vi "mod.Basic1.vi"(8 "error in":errorcluster, 11 "Call Data":T1) -> (0 "error out":errorcluster, 3 "Return Data":variant)   [LabVIEW 2014]
uses:
  Private/Class/typedef.LVCallData.ctl
  Private/Class/class.GLue.lvclass
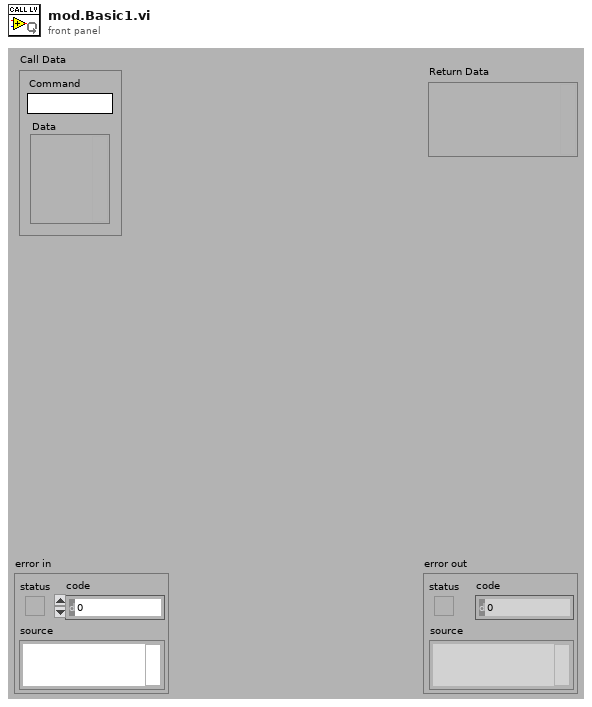
[diagram p1: front panel]
types:
  T1 = typedef "GLue.lvlib/class.GLue.lvclass/typedef.LVCallData.ctl" = cluster{"Command":string, "Data":variant}
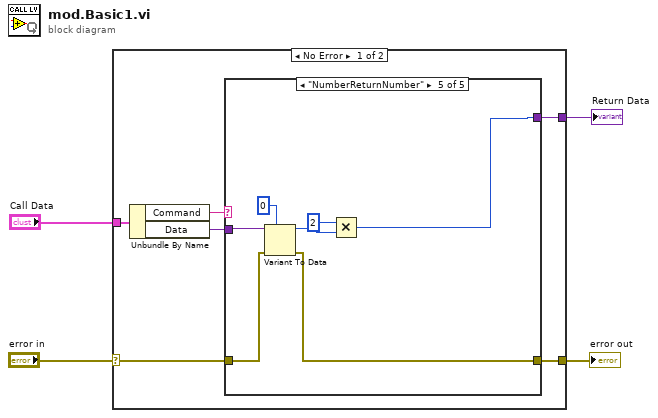
[diagram p0: block diagram]
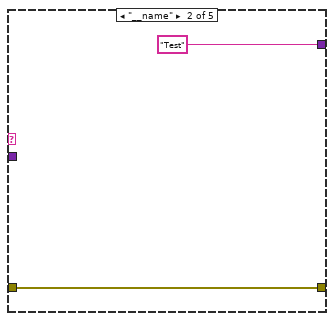
[diagram p3: hidden frame]
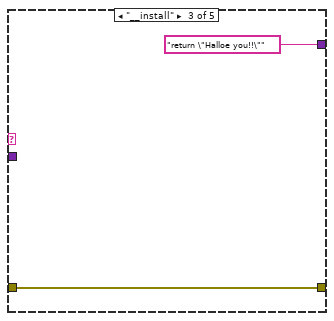
[diagram p4: hidden frame]
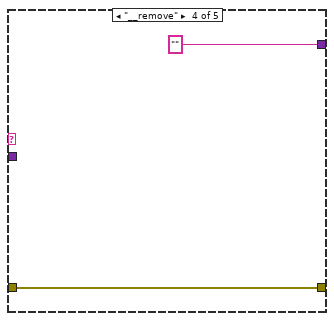
[diagram p5: hidden frame]
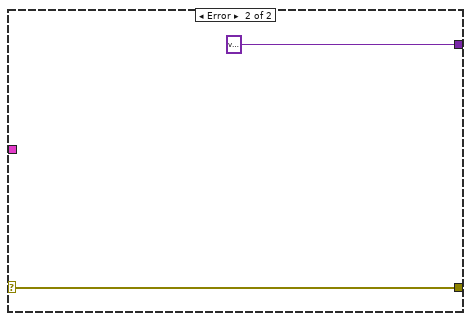
[diagram p6: hidden frame]
diagram:
  n1 = case shown="No Error" "error in" {
    selector: "error in" -> [w9 w27]
    tunnel: [w5 w27] -> w3
    tunnel: "Call Data" -> [w10 _]
    tunnel: [w6 variant ("User Data")] -> w1
    frame No Error {
      n2 = Unbundle By Name(w10) -> ("Command"=w8:string, "Data"=w7:variant)
      n3 = case shown="\"NumberReturnNumber\"" w8 {
        tunnel: w9 -> [w12 w13 w15 w17 w24]
        tunnel: w7 -> [w11 _ _ _ w25]
        tunnel: [w11 "Test" "return \"Halloe you!!\"" "" w20] -> w6
        tunnel: [w12 w13 w15 w17 w19] -> w5
        frame Default {
        }
        frame "__name" {
        }
        frame "__install" {
        }
        frame "__remove" {
        }
        frame "NumberReturnNumber" {
          n4 = Variant To Data(error in=w24, type=0, Variant=w25) -> (data=w22:i32, error out=w19:errorcluster)
          n5 = Multiply(x=2, y=w22) -> (x*y=w20:i32)
        }
      }
    }
    frame Error {
    }
  }
  "Return Data" <- w1
  "error out" <- w3
